vi "LoadingBar_General_UI.vi"(8 "error in (no error)":errorcluster, 10 "String\n to be displayed":string, 11 "Display?":bool) -> (0 "error out":errorcluster, 3 "Loading Bar VI\nRef":refnum<vi>)   [LabVIEW 2019, in "ZenGage v3.0 UI.lvclass"]
uses:
  ZenGage v3.0 UI.lvclass
panel:
  out "Displayed String":string
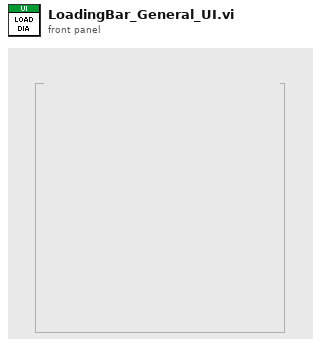
[diagram p1: front panel]
types:
  T1 = enum32{"Invalid", "Standard", "Closed", "Hidden", "Minimized", "Maximized"}
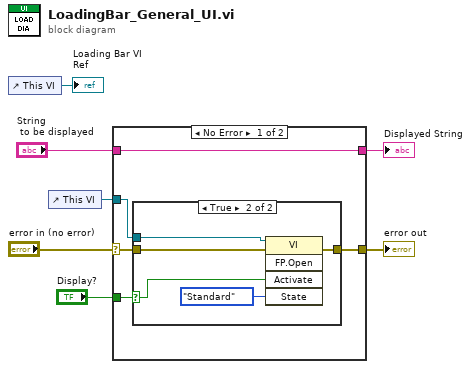
[diagram p0: block diagram]
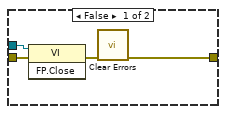
[diagram p2: hidden frame]
diagram:
  n1 = control-ref of="This VI"() -> (→"Loading Bar VI\nRef":refnum<vi>)
  n2 = control-ref of="This VI"() -> (w6:refnum<vi>)
  n3 = case shown="No Error" "error in (no error)" {
    selector: "error in (no error)" -> [w9 w23]
    tunnel: "Display?" -> [w12 _]
    tunnel: w6 -> [w11 _]
    tunnel: [w10 w23] -> w5
    tunnel: [w8 w22] -> w3
    tunnel: "String\n to be displayed" -> [w8 w22]
    frame No Error {
      n4 = case shown="True" w12 {
        selector: w12 -> [_ w20]
        tunnel: w11 -> [w15 w21]
        tunnel: w9 -> [w16 w19]
        tunnel: [w13 w18] -> w10
        frame False {
          n5 = invoke class="VI" method="FP.Close"(reference=w15, error in=w16) -> (error out=w14:errorcluster)  [unwired: 1 in, 2 out]
          n6 = call <vilib>:"Clear Errors.vi"("error in (no error)"=w14) -> ("error out"=w13:errorcluster)  [unwired: 5 in, 1 out]
        }
        frame True {
          n7 = invoke class="VI" method="FP.Open"(reference=w21, error in=w19, "Activate"=w20, "State"=T1."Standard") -> (error out=w18:errorcluster)  [unwired: 1 in, 4 out]
        }
      }
    }
    frame Error {
    }
  }
  "Displayed String" <- w3
  "error out" <- w5
